vi "PQfetchResultDataNotrans.vi"(8 "error in":errorcluster, 10 "res":u32, 11 "conn":u32) -> (0 "error out":errorcluster, 1 "Data":string[][](array[string]), 2 "res_out":u32, 3 "conn_out":u32, 4 "PQnFields":i32, 6 "PQnTuples":i32)   [LabVIEW 2019, in "libpqutility.lvlib"]
doc: "Fetch Result Data from DatabaseRequest into String Array.\nSee PostgreSQL c-lib doku for further information."
uses:
  libpqutility.lvlib
  libpqlv/libpqlv.lvlib
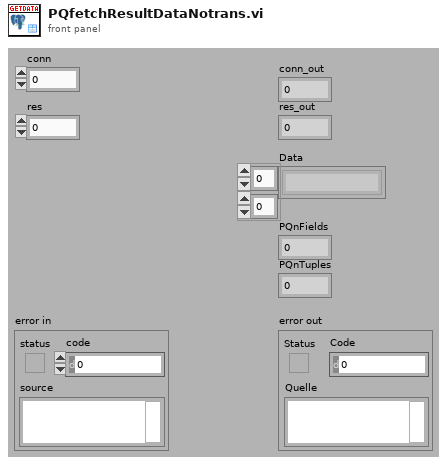
[diagram p1: front panel]
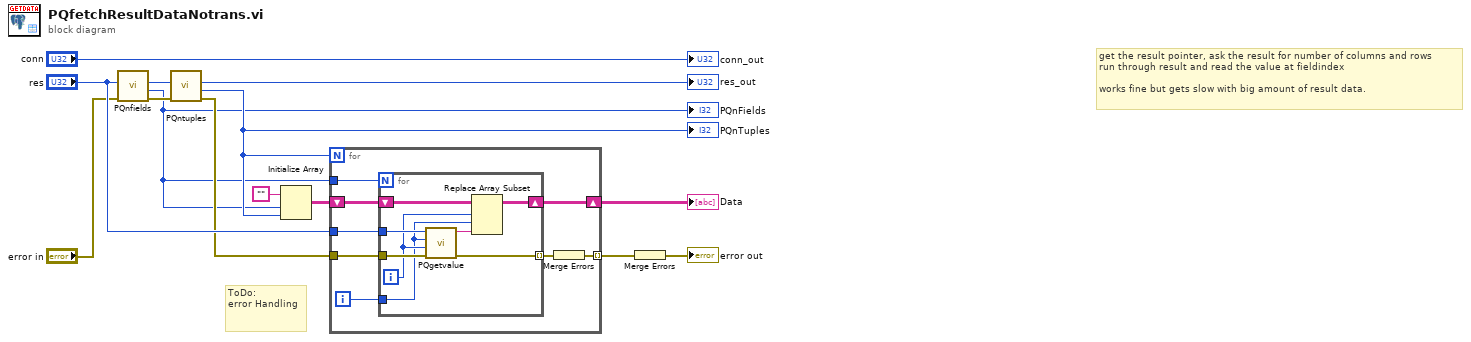
[diagram p0: block diagram]
diagram:
  # "ToDo:\nerror Handling"
  # "get the result pointer, ask the result for number of columns and rows\nrun through result and read the value at fieldindex\n\nworks fine but gets slow with big amount of result data."
  n1 = call "PQnfields.vi"("error in (no error)"="error in", "res"="res") -> ("error out"=w11:errorcluster, "PQnFields"=w1:i32, "res out"=w2:u32)  [unwired: 7 in]
  "PQnFields" <- w1
  n2 = call "PQntuples.vi"("error in (no error)"=w11, "res"=w2) -> ("error out"=w10:errorcluster, "PQnTuples"=w5:i32, "res out"=→"res_out":u32)  [unwired: 7 in]
  "PQnTuples" <- w5
  n3 = Initialize Array("", w1, w5) -> (w7:string[][])
  n4 = for {
    N: w5 -> [_]
    tunnel: "res" -> [w22]
    tunnel: w1 -> [w19]
    tunnel: w10 -> [w20]
    tunnel: [w15] -> w4 mode=indexing
    shift-right: [w18] -> w6
    shift-left: w7 -> [w17]
    i -> [w21]
    n5 = for {
      N: w19 -> [_]
      tunnel: w22 -> [w30]
      tunnel: w21 -> [w26]
      tunnel: w20 -> [w29]
      tunnel: [w28] -> w16 mode=indexing
      shift-right: [w24] -> w18
      shift-left: w17 -> [w23]
      i -> [w27]
      n6 = call "PQgetvalue.vi"("error in (no error)"=w29, "column_number"=w27, "row_number"=w26, "res"=w30) -> ("error out"=w28:errorcluster, "field_value"=w25:string)  [unwired: 6 in]
      n7 = Replace Array Subset(array=w23, new element=w25, index (row)=w27, index (col)=w26) -> (w24:string[][])
    }
    n8 = Merge Errors(w16) -> (w15:errorcluster)
  }
  "Data" <- w6
  n9 = Merge Errors(w4) -> (→"error out":errorcluster)
  "conn_out" <- "conn"
